vi "ImageArray2File (SubVI).vi"(5 "Array":dbl[][](array[numeric]), 7 "Save CSV Files Path":path, 8 "error in (no error)":errorcluster, 9 "Image file name ext":string, 10 "Image File Name":string, 11 "Content_ str":string) -> (0 "error out":errorcluster)   [LabVIEW 2016]
uses:
  <vilib>/Utility/file.llb/Write Delimited Spreadsheet (DBL).vi
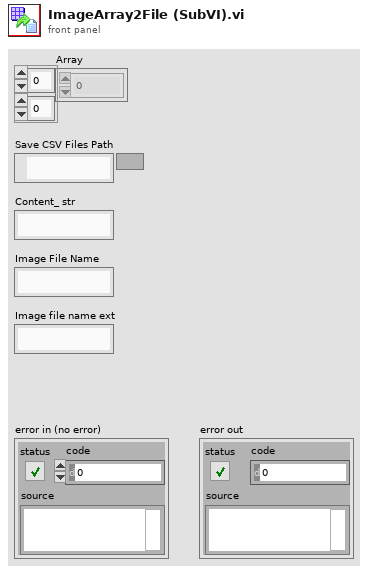
[diagram p1: front panel]
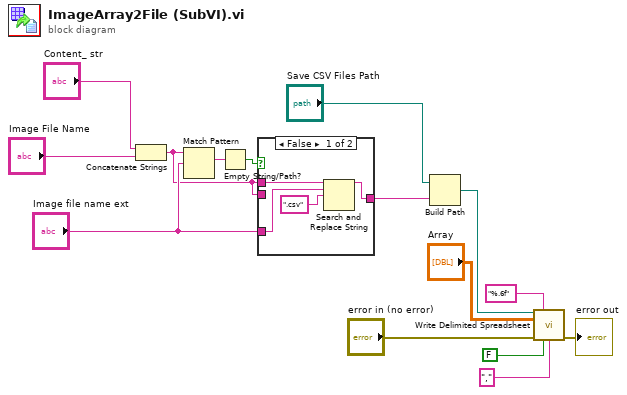
[diagram p0: block diagram]
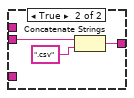
[diagram p2: hidden frame]
diagram:
  n1 = Concatenate Strings("Content_ str", "Image File Name") -> (w2:string)
  n2 = Match Pattern(string=w2, regular expression="Image file name ext") -> (match substring=w6:string)  [unwired: 1 in, 3 out]
  n3 = Empty String/Path?(string/path=w6) -> (empty?=w5:bool)
  n4 = case shown="False" w5 {
    tunnel: w2 -> [_ w22]
    tunnel: [w16 w20] -> w4
    tunnel: "Image file name ext" -> [w18 _]
    tunnel: w2 -> [w17 _]
    frame False {
      n5 = Search and Replace String(input string=w17, search string=w18, replace string=".csv" ("New ext for CSV")) -> (result string=w16:string)  [unwired: 5 in, 3 out]
    }
    frame True {
      n6 = Concatenate Strings(w22, ".csv" ("New ext for CSV")) -> (w20:string)
    }
  }
  n7 = Build Path(base path="Save CSV Files Path", name or relative path=w4) -> (appended path=w13:path)
  n8 = call-poly <vilib>:"Write Delimited Spreadsheet.vi"("file path (dialog if empty)"=w13, "format (%.3f)"="%.6f", "2D data"="Array", "error in (no error)"="error in (no error)", "transpose? (no:F)"=FALSE, "delimiter (\\t)"="," ("delimiter (\\t)")) -> ("error out"=→"error out":errorcluster)  [unwired: 8 in, 1 out]
